vi "Rtn Para Pwr Meas.vi"(6 "error in (no error)":errorcluster) -> (0 "error out":errorcluster, 3 "RtnParaPwr":T1)   [LabVIEW 2013, in "QCAWLAN_DLL.lvlib"]
doc: "QCA_DLL_Export void RtnParaPwrMeas(unsigned int* iGain, unsigned int* iFreq, double* dPowerLevel, unsigned int* iNumAvg, unsigned int* iTriggerType, int* iTriggerLevel, int* txChain);"
uses:
  QCAWLAN_DLL.lvlib
  QCAWLAN_DLL.dll
panel:
  in  "txChain":i32
  in  "iTriggerLevel":i32
  in  "iTriggerType":u32
  in  "iNumAvg":u32
  in  "dPowerLevel":dbl
  in  "iFreq":u32
  in  "iGain":u32
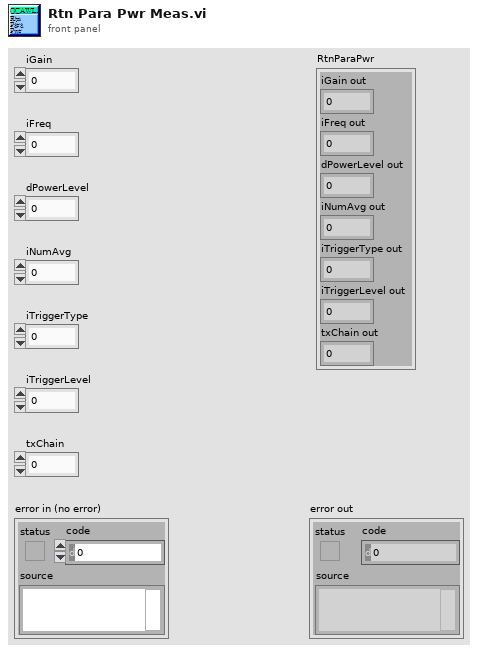
[diagram p1: front panel]
types:
  T1 = cluster{"iGain out":u32, "iFreq out":u32, "dPowerLevel out":dbl, "iNumAvg out":u32, "iTriggerType out":u32, "iTriggerLevel out":i32, "txChain out":i32}
  T2 = cluster{"iGain":u32, "iFreq":u32, "dPowerLevel":dbl, "iNumAvg":u32, "iTriggerType":u32, "iTriggerLevel":i32, "txChain":i32}
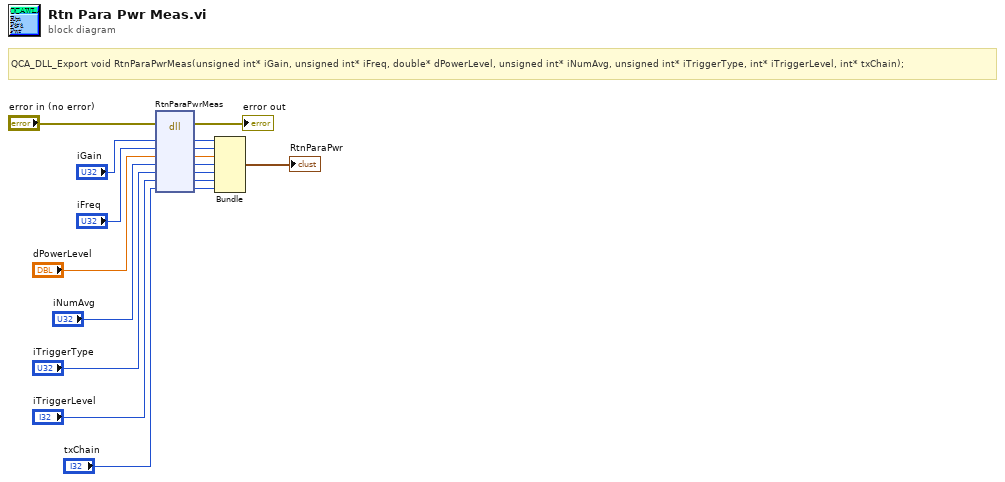
[diagram p0: block diagram]
diagram:
  # "QCA_DLL_Export void RtnParaPwrMeas(unsigned int* iGain, unsigned int* iFreq, double* dPowerLevel, unsigned int* iNumAvg, unsigned int* iTriggerType, int* iTriggerLevel, int* txChain);"
  n1 = dll-call lib="C:/Connectivity Client - MIMO/PlugIn/QCAWLAN_DLL.dll" fn="RtnParaPwrMeas"(error in="error in (no error)", "iGain"="iGain", "iFreq"="iFreq", "dPowerLevel"="dPowerLevel", "iNumAvg"="iNumAvg", "iTriggerType"="iTriggerType", "iTriggerLevel"="iTriggerLevel", "txChain"="txChain") -> (error out=→"error out":errorcluster, "iGain"=w8:u32, "iFreq"=w7:u32, "dPowerLevel"=w6:dbl, "iNumAvg"=w5:u32, "iTriggerType"=w4:u32, "iTriggerLevel"=w3:i32, "txChain"=w2:i32)  [unwired: 3 in, 1 out]
  n2 = Bundle("iGain"=w8, "iFreq"=w7, "dPowerLevel"=w6, "iNumAvg"=w5, "iTriggerType"=w4, "iTriggerLevel"=w3, "txChain"=w2) -> (→"RtnParaPwr":T2)  [unwired: 1 in]
